vi "step function (SubVI).vi"(1 "input":dbl) -> (0 "output":dbl)   [LabVIEW 2023]
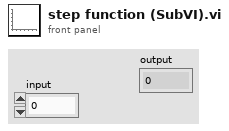
[diagram p1: front panel]
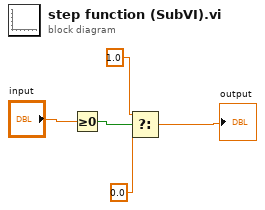
[diagram p0: block diagram]
diagram:
  n1 = Greater Or Equal To 0?(x="input") -> (x >= 0?=w1:bool)
  n2 = Select(t=1.0, s=w1, f=0.0) -> (s? t:f=→"output":dbl)
